vi "Defragment is in Progress.vi"(8 "error in (no error)":errorcluster) -> (0 "error out":errorcluster, 4 "This VI":refnum<vi>)   [LabVIEW 2014]
doc: "<B>Copyright</B>: (c) MHWirth 2015. All rights reserved."
panel:
  # "Defragmentation in progress ..."
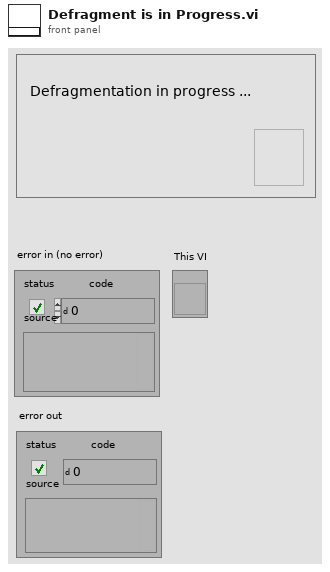
[diagram p1: front panel]
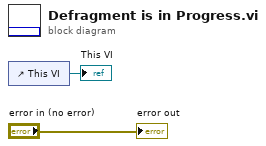
[diagram p0: block diagram]
diagram:
  n1 = control-ref of="This VI"() -> (→"This VI":refnum<vi>)
  "error out" <- "error in (no error)"
